vi "ZVL Network Analyser - send GPIB cmd.vi"(8 "error in (no error)":errorcluster, 10 "Cmd string":string="power -10 0") -> (0 "error out":errorcluster, 2 "Response":string)   [LabVIEW 2019]
doc: "Nicolas Weiss - EPFL - IPHYS 2019\n----\nThis VI sends the GPIB commands to the device (without performing syntax and in-range argument check).\nThus, the commands *must* first be checked by the \"Check and send command to corresponding device.vi\""
uses:
  _Global variables 1.vi
  <instrlib>/rszvl/_utility/rsidr_core.llb/rszvl_rsidr_core.lvlib
panel:
  out "Arguments":string[](array[string])
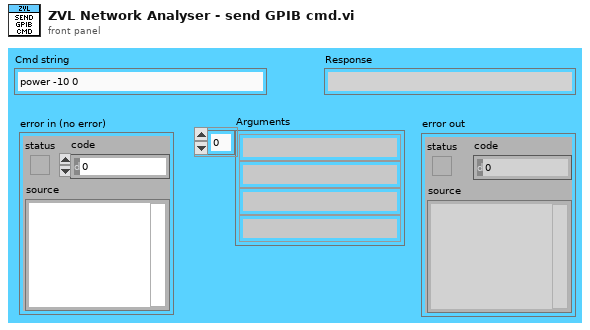
[diagram p1: front panel]
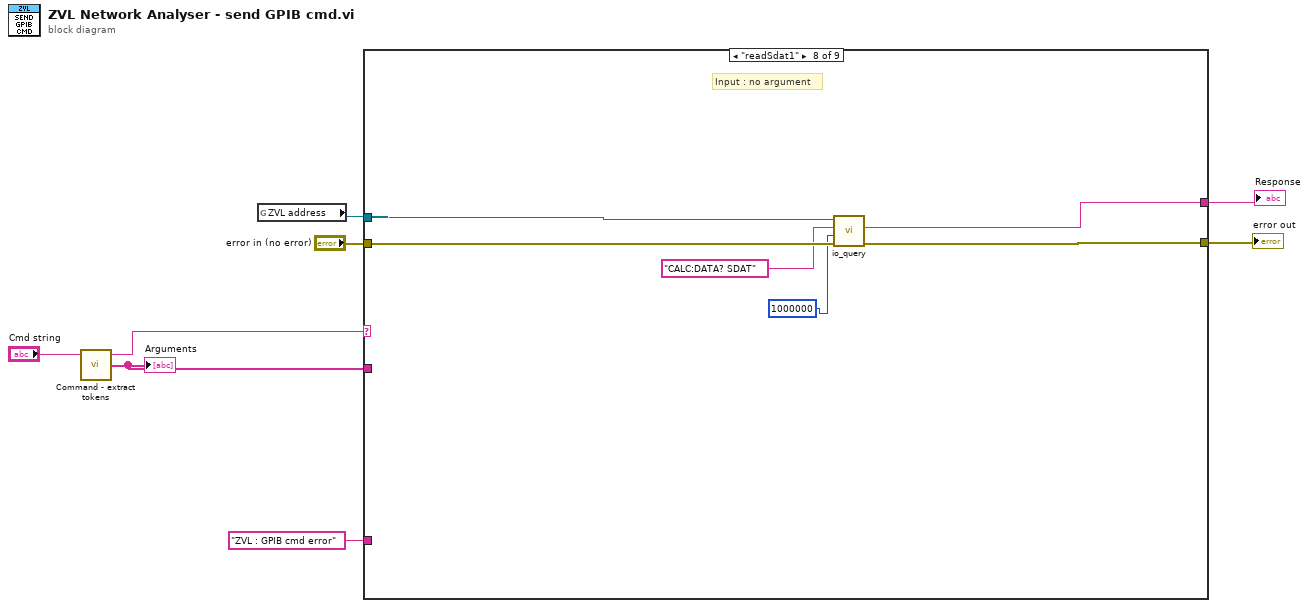
[diagram p0: block diagram]
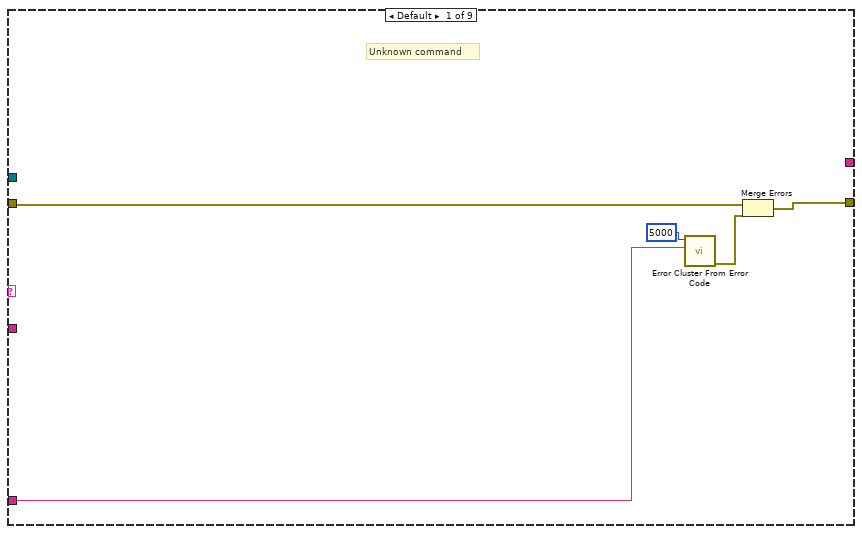
[diagram p2: hidden frame]
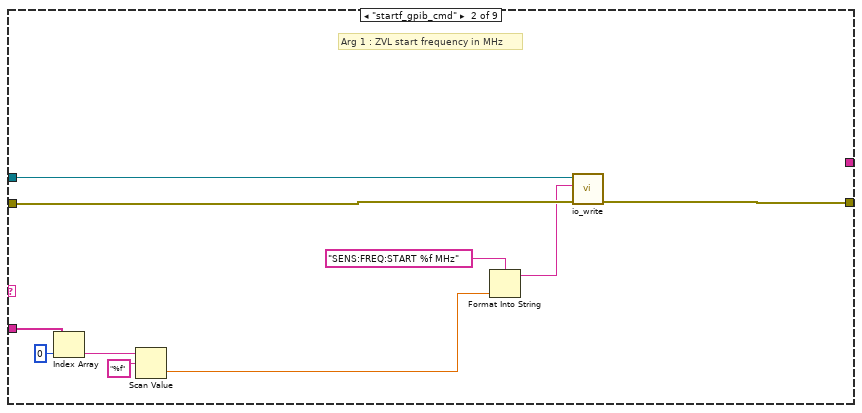
[diagram p3: hidden frame]
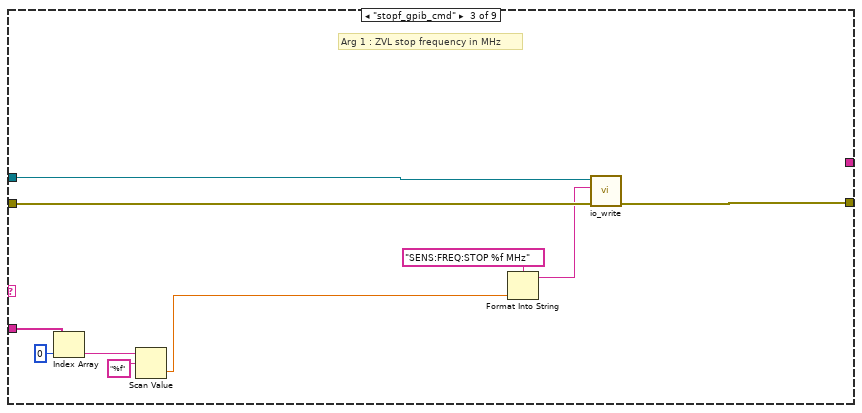
[diagram p4: hidden frame]
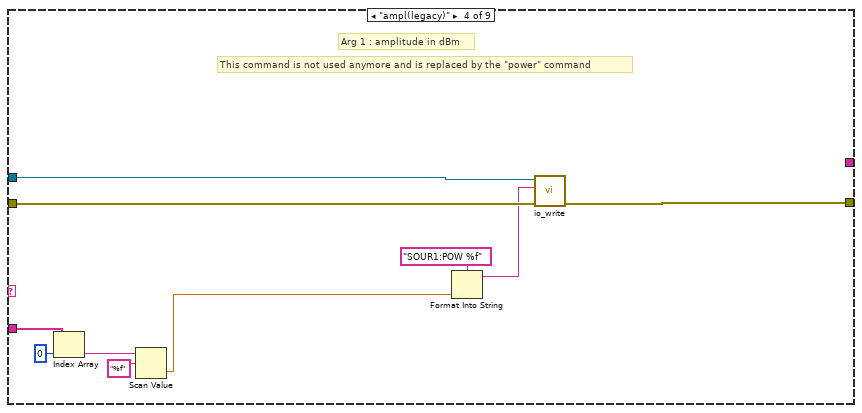
[diagram p5: hidden frame]
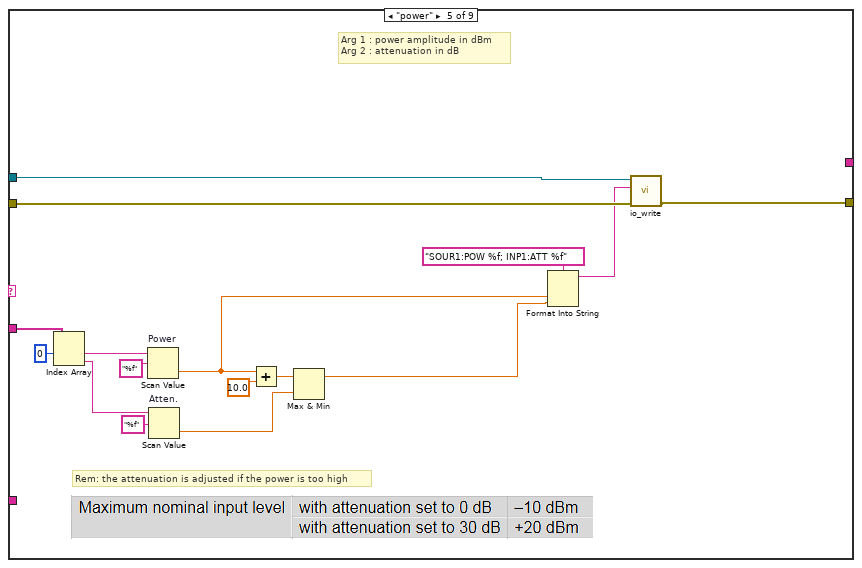
[diagram p6: hidden frame]
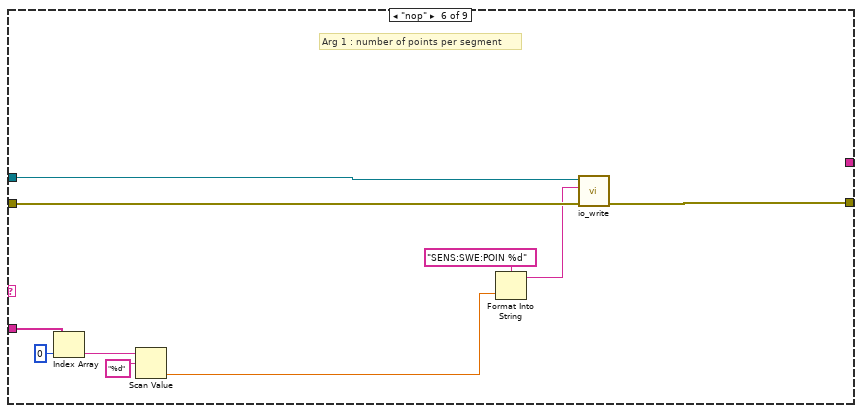
[diagram p7: hidden frame]
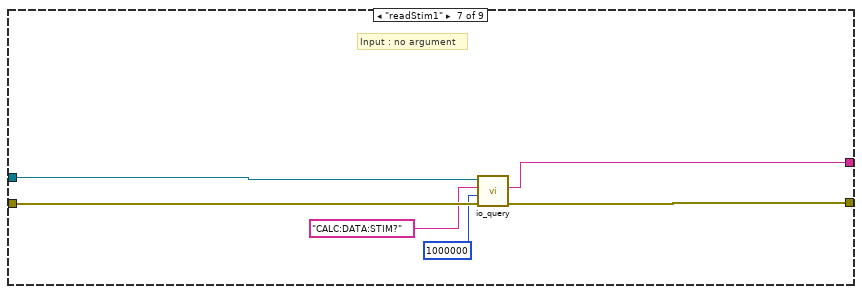
[diagram p8: hidden frame]
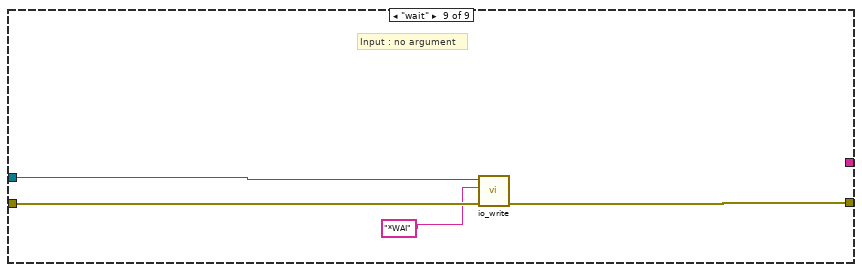
[diagram p9: hidden frame]
diagram:
  n1 = call "Command - extract tokens.vi"("Cmd string"="Cmd string") -> ("Arguments"=w3:string[], "Command"=w1:string)  [unwired: 2 in, 1 out]
  "Arguments" <- w3
  n2 = global read "_Global variables 1.vi" "ZVL address"() -> (w5:refnum<visa-resource-name>)
  n3 = case shown="\"readSdat1\"" w1 {
    tunnel: w3 -> [_ w21 w31 w41 w58 w67 _ _ _]
    tunnel: w5 -> [_ w19 w29 w39 w56 w65 w73 w79 w85]
    tunnel: "error in (no error)" -> [w10 w17 w27 w37 w55 w63 w74 w80 w84]
    tunnel: [w11 w16 w26 w36 w54 w62 w75 w81 w83] -> w7
    tunnel: [_ _ _ _ _ _ w72 w77 _] -> w6
    tunnel: "ZVL : GPIB cmd error" ("format string") -> [w9 _ _ _ _ _ _ _ _]
    frame Default {
      # "Unknown command"
      n4 = call <vilib>:"Error Cluster From Error Code.vi"("error message (\"\")"=w9, "error code (0)"=5000) -> ("error out"=w13:errorcluster)  [unwired: 7 in]
      n5 = Merge Errors(w10, w13) -> (w11:errorcluster)
    }
    frame "startf_gpib_cmd" {
      # "Arg 1 : ZVL start frequency in MHz"
      n6 = Index Array(array=w21, index=0) -> (element=w20:string)
      n7 = Scan Value(string=w20, format string="%f") -> (value=w18:dbl)  [unwired: 1 in, 1 out]
      n8 = Format Into String(format string="SENS:FREQ:START %f MHz", w18) -> (resulting string=w15:string)  [unwired: 2 in, 1 out]
      n9 = call <instrlib>:"io_write.vi"("error in"=w17, "write buffer"=w15, "VISA resource name"=w19) -> ("error out"=w16:errorcluster)  [unwired: 7 in, 1 out]
    }
    frame "stopf_gpib_cmd" {
      # "Arg 1 : ZVL stop frequency in MHz"
      n10 = Index Array(array=w31, index=0) -> (element=w30:string)
      n11 = Scan Value(string=w30, format string="%f") -> (value=w28:dbl)  [unwired: 1 in, 1 out]
      n12 = Format Into String(format string="SENS:FREQ:STOP %f MHz", w28) -> (resulting string=w25:string)  [unwired: 2 in, 1 out]
      n13 = call <instrlib>:"io_write.vi"("error in"=w27, "write buffer"=w25, "VISA resource name"=w29) -> ("error out"=w26:errorcluster)  [unwired: 7 in, 1 out]
    }
    frame "ampl(legacy)" {
      # "This command is not used anymore and is replaced by the \"power\" command"
      # "Arg 1 : amplitude in dBm"
      n14 = Index Array(array=w41, index=0) -> (element=w40:string)
      n15 = Scan Value(string=w40, format string="%f") -> (value=w38:dbl)  [unwired: 1 in, 1 out]
      n16 = Format Into String(format string="SOUR1:POW %f", w38) -> (resulting string=w34:string)  [unwired: 2 in, 1 out]
      n17 = call <instrlib>:"io_write.vi"("error in"=w37, "write buffer"=w34, "VISA resource name"=w39) -> ("error out"=w36:errorcluster)  [unwired: 7 in, 1 out]
    }
    frame "power" {
      # "Rem: the attenuation is adjusted if the power is too high"
      # "Arg 1 : power amplitude in dBm\nArg 2 : attenuation in dB"
      n18 = Index Array(array=w58, index #1=0 ("index")) -> (element #1=w57:string, element #2=w51:string)  [unwired: 1 in]
      n19 = Scan Value "Power"(string=w57, format string="%f") -> (value=w48:dbl)  [unwired: 1 in, 1 out]
      n20 = Scan Value "Atten."(string=w51, format string="%f") -> (value=w46:dbl)  [unwired: 1 in, 1 out]
      n21 = Add(x=w48, y=10.0) -> (x+y=w47:dbl)
      n22 = Max & Min(x=w47, y=w46) -> (max(x,y)=w45:dbl)  [unwired: 1 out]
      n23 = Format Into String(format string="SOUR1:POW %f; INP1:ATT %f", w48, w45) -> (resulting string=w52:string)  [unwired: 2 in, 1 out]
      n24 = call <instrlib>:"io_write.vi"("error in"=w55, "write buffer"=w52, "VISA resource name"=w56) -> ("error out"=w54:errorcluster)  [unwired: 7 in, 1 out]
    }
    frame "nop" {
      # "Arg 1 : number of points per segment"
      n25 = Index Array(array=w67, index=0) -> (element=w66:string)
      n26 = Scan Value(string=w66, format string="%d") -> (value=w64:dbl)  [unwired: 1 in, 1 out]
      n27 = Format Into String(format string="SENS:SWE:POIN %d", w64) -> (resulting string=w61:string)  [unwired: 2 in, 1 out]
      n28 = call <instrlib>:"io_write.vi"("error in"=w63, "write buffer"=w61, "VISA resource name"=w65) -> ("error out"=w62:errorcluster)  [unwired: 7 in, 1 out]
    }
    frame "readStim1" {
      # "Input : no argument"
      n29 = call <instrlib>:"io_query.vi"("error in"=w74, "Bytes to read (2048)"=u32 1000000, "write buffer"="CALC:DATA:STIM?" ("format string"), "VISA resource name"=w73) -> ("error out"=w75:errorcluster, "read buffer"=w72:string)  [unwired: 4 in, 2 out]
    }
    frame "readSdat1" {
      # "Input : no argument"
      n30 = call <instrlib>:"io_query.vi"("error in"=w80, "Bytes to read (2048)"=u32 1000000, "write buffer"="CALC:DATA? SDAT" ("format string"), "VISA resource name"=w79) -> ("error out"=w81:errorcluster, "read buffer"=w77:string)  [unwired: 4 in, 2 out]
    }
    frame "wait" {
      # "Input : no argument"
      n31 = call <instrlib>:"io_write.vi"("error in"=w84, "write buffer"="*WAI" ("format string"), "VISA resource name"=w85) -> ("error out"=w83:errorcluster)  [unwired: 7 in, 1 out]
    }
  }
  "error out" <- w7
  "Response" <- w6
